vi "TestExec.Config, Get Barcode PN SN Format Info.vi"(8 "error in":errorcluster, 11 "Config File":path) -> (0 "error out":errorcluster, 3 "Barcode PN SN Format":T1={"Type"=enum."SN_Only", "Len"=12, "Delimiter"="TAB"})   [LabVIEW 2018]
uses:
  Controls and Type Defs/TestExec.Barcode PN SN Format Type.ctl
  <vilib>/Utility/config.llb/Read Key (String).vi
  <vilib>/Utility/config.llb/Read Key (I32).vi
  <vilib>/Utility/config.llb/NI_LVConfig.lvlib
  <vilib>/KATE/Files/File Utils.lvlib
panel:
  # "String or Special Chars: \n  TAB CR LF EOL(CRLF)"
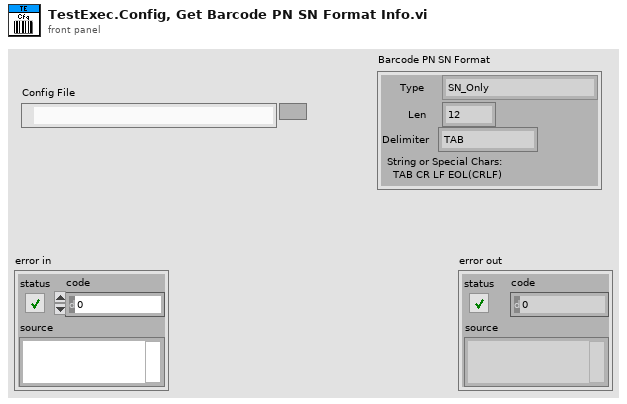
[diagram p1: front panel]
types:
  T1 = typedef "TestExec.Barcode PN SN Format Type.ctl" = cluster{"Type":enum16{"SN_Only", "SN_PN_LenDelim", "PN_SN_LenDelim", "SN_PN_StrDelim", "PN_SN_StrDelim"}, "Len":i32, "Delimiter":string}
  T2 = enum16{"SN_Only", "SN_PN_LenDelim", "PN_SN_LenDelim", "SN_PN_StrDelim", "PN_SN_StrDelim"}
  T3 = typedef "NI_LVConfig.lvlib/Config Data RefNum.ctl" = refnum<k1>
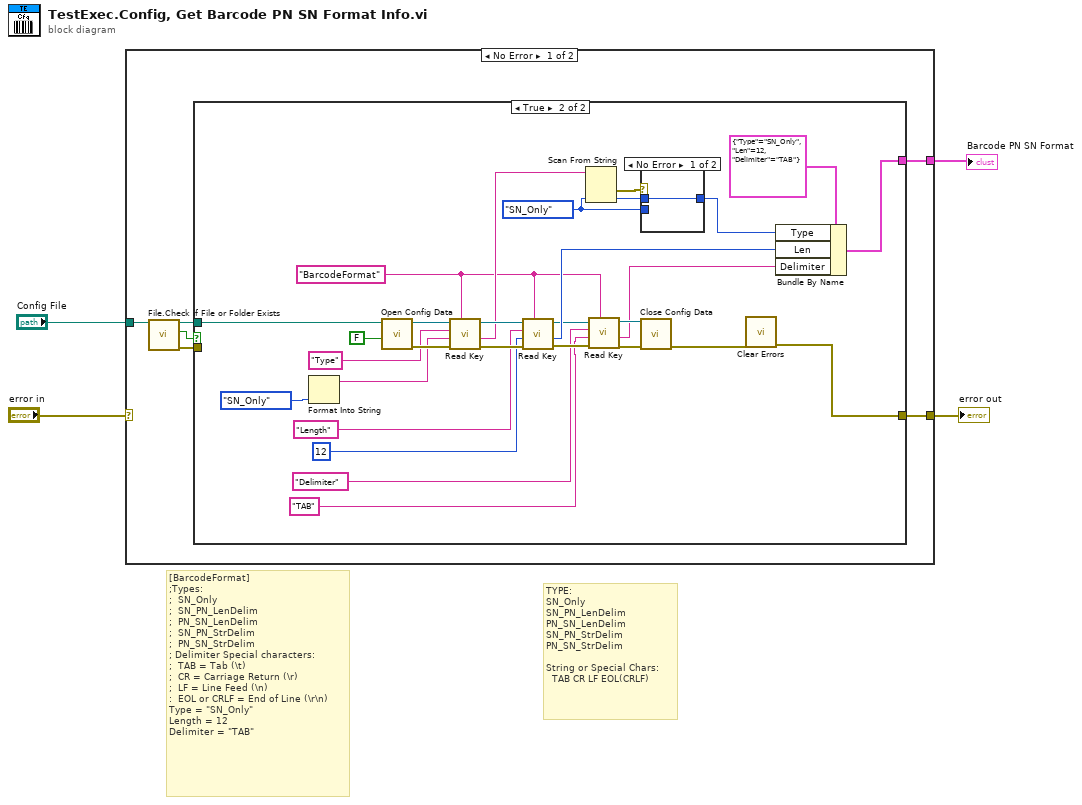
[diagram p0: block diagram]
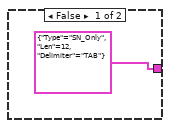
[diagram p2: hidden frame]
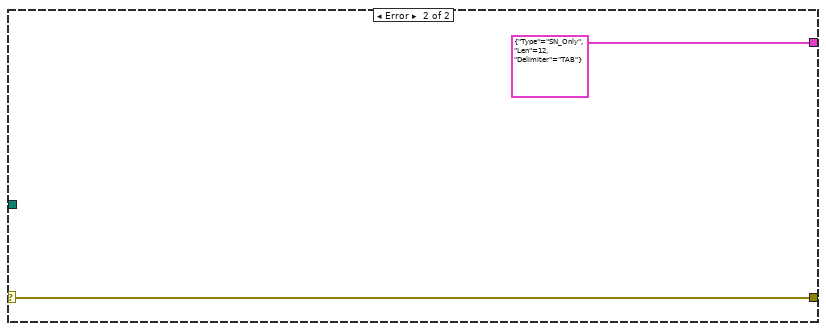
[diagram p4: hidden frame]
diagram:
  # "[BarcodeFormat]\n;Types:\n;  SN_Only\n;  SN_PN_LenDelim\n;  PN_SN_LenDelim\n;  SN_PN_StrDelim\n;  PN_SN_StrDelim\n; Delimiter Special characters:\n;  TAB = Tab (\\t)\n;  CR = Carriage Return (\\r)\n;  LF = Line Feed (\\n)\n:  EOL or CRLF = End of Line (\\r\\n)\nType = \"SN_Only\"\nLength = 12\nDelimiter = \"TAB\""
  # "TYPE:\nSN_Only\nSN_PN_LenDelim\nPN_SN_LenDelim\nSN_PN_StrDelim\nPN_SN_StrDelim\n\nString or Special Chars: \n  TAB CR LF EOL(CRLF)"
  n1 = case shown="No Error" "error in" {
    selector: "error in" -> [_ w44]
    tunnel: [w10 w44] -> w3
    tunnel: [w9 T1 {"Type"=enum."SN_Only", "Len"=12, "Delimiter"="TAB"} ("Barcode PN SN Format")] -> w2
    tunnel: "Config File" -> [w8 _]
    frame No Error {
      n2 = call <vilib>:"File.Check if File or Folder Exists.vi"("Path"=w8) -> ("error out"=w5:errorcluster, "Exists"=w6:bool, "Dup Path"=w7:path)  [unwired: 6 in, 2 out]
      n3 = case shown="True" w6 {
        tunnel: [_ w31] -> w10
        tunnel: [T1 {"Type"=enum."SN_Only", "Len"=12, "Delimiter"="TAB"} ("Barcode PN SN Format") w24] -> w9
        tunnel: w7 -> [_ w12]
        tunnel: w5 -> [_ _]
        frame False {
        }
        frame True {
          w17 = T2."SN_Only" ("Type")
          w14 = "BarcodeFormat"
          n4 = Format Into String(T2."SN_Only" ("Type")) -> (resulting string=w21:string)  [unwired: 3 in, 1 out]
          n5 = call <vilib>:"Open Config Data.vi"("create file if necessary (T)"=FALSE, "configuration file path"=w12) -> ("error out"=w39:errorcluster, "refnum"=w40:T3)  [unwired: 7 in, 1 out]
          n6 = call-poly <vilib>:"Read Key.vi"("section"=w14, "error in (no error)"=w39, "default value"=w21, "key"="Type", "refnum"=w40) -> ("error out"=w35:errorcluster, "value"=w16:string, "refnum out"=w36:T3)  [unwired: 3 in, 1 out]
          n7 = call-poly <vilib>:"Read Key.vi"("section"=w14, "error in (no error)"=w35, "default value"=12 ("Len"), "key"="Length", "refnum"=w36) -> ("error out"=w27:errorcluster, "value"=w32:i32, "refnum out"=w30:T3)  [unwired: 3 in, 1 out]
          n8 = Scan From String(input string=w16, default 1=w17) -> (error out=w18:errorcluster, output 1=w19:T2)  [unwired: 3 in, 2 out]
          n9 = call-poly <vilib>:"Read Key.vi"("section"=w14, "error in (no error)"=w27, "default value"="TAB", "key"="Delimiter", "refnum"=w30) -> ("error out"=w28:errorcluster, "value"=w25:string, "refnum out"=w29:T3)  [unwired: 3 in, 1 out]
          n10 = case shown="No Error" w18 {
            tunnel: w17 -> [_ w42]
            tunnel: w19 -> [w41 _]
            tunnel: [w41 w42] -> w15
            frame No Error {
            }
            frame Error {
            }
          }
          n11 = call <vilib>:"Close Config Data.vi"("error in (no error)"=w28, "refnum"=w29) -> ("error out"=w37:errorcluster)  [unwired: 8 in, 1 out]
          n12 = call <vilib>:"Clear Errors.vi"("error in (no error)"=w37) -> ("error out"=w31:errorcluster)  [unwired: 5 in, 1 out]
          n13 = Bundle By Name(cluster=T1 {"Type"=enum."SN_Only", "Len"=12, "Delimiter"="TAB"} ("Barcode PN SN Format"), "Type"=w15, "Len"=w32, "Delimiter"=w25) -> (w24:T1)
        }
      }
    }
    frame Error {
    }
  }
  "error out" <- w3
  "Barcode PN SN Format" <- w2
